vi "main(Test DQMH modules).bak.vi"() -> ()   [LabVIEW 2018, in "Application.lvlib"] (continued)
        n3308 = Bundle By Name(cluster=w7269, "command"="MEAS.eMIC", "command data"=w7266) -> (w7261:T11)
        n3309 = Bundle By Name(cluster=w7269, "command"="MEAS.AllRelaysOFF") -> (w7265:T11)
        n3310 = Build Array(w7265, w7264, w7263, w7262, w7261) -> (w7256:T11[])
        n3311 = Bundle By Name(cluster=w7243, "command"="MEAS.requestAC", "command data"=w7236) -> (w7257:T11)
        n3312 = Bundle By Name(cluster=w7243, "command"="Apps.WaitForEvent", "command data"=w7236) -> (w7242:T11)
        n3313 = Bundle By Name(cluster=w7243, "command"="MEAS.DMM dual read") -> (w7258:T11)
        n3314 = Bundle By Name(cluster=w7243, "command"="Apps.UI Update 1") -> (w7244:T11)
        n3315 = Build Array(w7258, w7257, w7242, w7244) -> (w7255:T11[])
        n3316 = Build Array (concatenate)(w7256, w7255) -> (w7254:T11[])
        n3317 = for {
          tunnel: w7254 -> [w7291] mode=indexing
          tunnel: w7249 -> [w7292]
          tunnel: [w7288] -> w7252 mode=indexing
          n3318 = Unbundle By Name(w7291) -> ("command"=w7290:string, "command data"=w7289:variant)
          n3319 = call "App enquece.vi"("command data"=w7289, "command"=w7290, "queue in"=w7292) -> ("error out"=w7288:errorcluster)  [unwired: 7 in, 1 out]
        }
        n3320 = Merge Errors(w7253, w7252) -> (w7251:errorcluster)
      }
      frame "Test DRV 29A" {
        w7300 = T11 {"command"="", "command data"=variant} ("element")
        w7294 = 29 ("DUT index(0-59)")
        w7326 = T11 {"command"="", "command data"=variant} ("element")
        n3321 = disable-structure shown="LOGGING==TRUE" {
          disable-tunnel: w7304 -> [w7341 _]
          frame condition #0 (active) {
            n3322 = Empty String/Path?(string/path=w7341) -> (empty?=w7344:bool)
            n3323 = Select(t="Quece timeout", s=w7344, f=w7341) -> (s? t:f=w7340:string)
            n3324 = call "string log (SubVI).vi"("Enum"=enum16{"Init", "Log", "Read"}."Log", "state Name"=w7340) -> ()  [unwired: 8 in, 2 out]
          }
          frame condition #1 {
          }
        }
        n3325 = Flush Queue(queue=w7305) -> (queue out=w7306:refnum<queue>)  [unwired: 1 in, 2 out]
        n3326 = Decrement(x=w7294) -> (x-1=w7297:i32)
        n3327 = Index Array(array=w7293, index=w7297) -> (element=w7295:refnum<vi>)
        n3328 = property class="ColBox"(reference=w7295, "Value"=u32 10000536 ("DRV 1")) -> ()  [unwired: 1 in, 2 out]
        n3329 = To Variant(anything=bool[] [FALSE, FALSE, FALSE, FALSE, TRUE, FALSE]) -> (Variant=w7323:variant)
        n3330 = To Variant(anything=T6."demux1_10_channel5" ("demux1_10(x6)_encode")) -> (Variant=w7327:variant)
        n3331 = To Variant(anything=T4."mux6_1_channel5_3" ("mux6_1(3wires)_encode")) -> (Variant=w7330:variant)
        n3332 = To Variant(anything=T5."mux10_1_channel5" ("mux10_1(x6)_encode")) -> (Variant=w7332:variant)
        n3333 = Bundle By Name(cluster=w7326, "command"="MEAS.mux10-1", "command data"=w7332) -> (w7321:T11)
        n3334 = Bundle By Name(cluster=w7326, "command"="MEAS.mux6_1", "command data"=w7330) -> (w7320:T11)
        n3335 = Bundle By Name(cluster=w7326, "command"="MEAS.demux1-10", "command data"=w7327) -> (w7319:T11)
        n3336 = Bundle By Name(cluster=w7326, "command"="MEAS.eMIC", "command data"=w7323) -> (w7318:T11)
        n3337 = Bundle By Name(cluster=w7326, "command"="MEAS.AllRelaysOFF") -> (w7322:T11)
        n3338 = Build Array(w7322, w7321, w7320, w7319, w7318) -> (w7313:T11[])
        n3339 = Bundle By Name(cluster=w7300, "command"="MEAS.requestAC", "command data"=w7294) -> (w7314:T11)
        n3340 = Bundle By Name(cluster=w7300, "command"="Apps.WaitForEvent", "command data"=w7294) -> (w7299:T11)
        n3341 = Bundle By Name(cluster=w7300, "command"="MEAS.DMM dual read") -> (w7315:T11)
        n3342 = Bundle By Name(cluster=w7300, "command"="Apps.UI Update 1") -> (w7301:T11)
        n3343 = Build Array(w7315, w7314, w7299, w7301) -> (w7312:T11[])
        n3344 = Build Array (concatenate)(w7313, w7312) -> (w7311:T11[])
        n3345 = for {
          tunnel: w7311 -> [w7348] mode=indexing
          tunnel: w7306 -> [w7349]
          tunnel: [w7345] -> w7309 mode=indexing
          n3346 = Unbundle By Name(w7348) -> ("command"=w7347:string, "command data"=w7346:variant)
          n3347 = call "App enquece.vi"("command data"=w7346, "command"=w7347, "queue in"=w7349) -> ("error out"=w7345:errorcluster)  [unwired: 7 in, 1 out]
        }
        n3348 = Merge Errors(w7310, w7309) -> (w7308:errorcluster)
      }
      frame "Test DRV 30A" {
        w7357 = T11 {"command"="", "command data"=variant} ("element")
        w7350 = 30 ("DUT index(0-59)")
        w7383 = T11 {"command"="", "command data"=variant} ("element")
        n3349 = disable-structure shown="LOGGING==TRUE" {
          disable-tunnel: w7361 -> [w7398 _]
          frame condition #0 (active) {
            n3350 = Empty String/Path?(string/path=w7398) -> (empty?=w7401:bool)
            n3351 = Select(t="Quece timeout", s=w7401, f=w7398) -> (s? t:f=w7397:string)
            n3352 = call "string log (SubVI).vi"("Enum"=enum16{"Init", "Log", "Read"}."Log", "state Name"=w7397) -> ()  [unwired: 8 in, 2 out]
          }
          frame condition #1 {
          }
        }
        n3353 = Flush Queue(queue=w7362) -> (queue out=w7363:refnum<queue>)  [unwired: 1 in, 2 out]
        n3354 = Decrement(x=w7350) -> (x-1=w7354:i32)
        n3355 = Index Array(array=w7351, index=w7354) -> (element=w7352:refnum<vi>)
        n3356 = property class="ColBox"(reference=w7352, "Value"=u32 10000536 ("DRV 1")) -> ()  [unwired: 1 in, 2 out]
        n3357 = To Variant(anything=bool[] [FALSE, FALSE, FALSE, FALSE, FALSE, TRUE]) -> (Variant=w7380:variant)
        n3358 = To Variant(anything=T6."demux1_10_channel5" ("demux1_10(x6)_encode")) -> (Variant=w7384:variant)
        n3359 = To Variant(anything=T4."mux6_1_channel6_3" ("mux6_1(3wires)_encode")) -> (Variant=w7387:variant)
        n3360 = To Variant(anything=T5."mux10_1_channel5" ("mux10_1(x6)_encode")) -> (Variant=w7389:variant)
        n3361 = Bundle By Name(cluster=w7383, "command"="MEAS.mux10-1", "command data"=w7389) -> (w7378:T11)
        n3362 = Bundle By Name(cluster=w7383, "command"="MEAS.mux6_1", "command data"=w7387) -> (w7377:T11)
        n3363 = Bundle By Name(cluster=w7383, "command"="MEAS.demux1-10", "command data"=w7384) -> (w7376:T11)
        n3364 = Bundle By Name(cluster=w7383, "command"="MEAS.eMIC", "command data"=w7380) -> (w7375:T11)
        n3365 = Bundle By Name(cluster=w7383, "command"="MEAS.AllRelaysOFF") -> (w7379:T11)
        n3366 = Build Array(w7379, w7378, w7377, w7376, w7375) -> (w7370:T11[])
        n3367 = Bundle By Name(cluster=w7357, "command"="MEAS.requestAC", "command data"=w7350) -> (w7371:T11)
        n3368 = Bundle By Name(cluster=w7357, "command"="Apps.WaitForEvent", "command data"=w7350) -> (w7356:T11)
        n3369 = Bundle By Name(cluster=w7357, "command"="MEAS.DMM dual read") -> (w7372:T11)
        n3370 = Bundle By Name(cluster=w7357, "command"="Apps.UI Update 1") -> (w7358:T11)
        n3371 = Build Array(w7372, w7371, w7356, w7358) -> (w7369:T11[])
        n3372 = Build Array (concatenate)(w7370, w7369) -> (w7368:T11[])
        n3373 = for {
          tunnel: w7368 -> [w7405] mode=indexing
          tunnel: w7363 -> [w7406]
          tunnel: [w7402] -> w7366 mode=indexing
          n3374 = Unbundle By Name(w7405) -> ("command"=w7404:string, "command data"=w7403:variant)
          n3375 = call "App enquece.vi"("command data"=w7403, "command"=w7404, "queue in"=w7406) -> ("error out"=w7402:errorcluster)  [unwired: 7 in, 1 out]
        }
        n3376 = Merge Errors(w7367, w7366) -> (w7365:errorcluster)
      }
      frame "Test DRV 31A" {
        w7414 = T11 {"command"="", "command data"=variant} ("element")
        w7407 = 31 ("DUT index(0-59)")
        w7440 = T11 {"command"="", "command data"=variant} ("element")
        n3377 = disable-structure shown="LOGGING==TRUE" {
          disable-tunnel: w7418 -> [w7455 _]
          frame condition #0 (active) {
            n3378 = Empty String/Path?(string/path=w7455) -> (empty?=w7458:bool)
            n3379 = Select(t="Quece timeout", s=w7458, f=w7455) -> (s? t:f=w7454:string)
            n3380 = call "string log (SubVI).vi"("Enum"=enum16{"Init", "Log", "Read"}."Log", "state Name"=w7454) -> ()  [unwired: 8 in, 2 out]
          }
          frame condition #1 {
          }
        }
        n3381 = Flush Queue(queue=w7419) -> (queue out=w7420:refnum<queue>)  [unwired: 1 in, 2 out]
        n3382 = Decrement(x=w7407) -> (x-1=w7411:i32)
        n3383 = Index Array(array=w7408, index=w7411) -> (element=w7409:refnum<vi>)
        n3384 = property class="ColBox"(reference=w7409, "Value"=u32 10000536 ("DRV 1")) -> ()  [unwired: 1 in, 2 out]
        n3385 = To Variant(anything=bool[] [TRUE, FALSE, FALSE, FALSE, FALSE, FALSE]) -> (Variant=w7437:variant)
        n3386 = To Variant(anything=T6."demux1_10_channel6" ("demux1_10(x6)_encode")) -> (Variant=w7441:variant)
        n3387 = To Variant(anything=T4."mux6_1_channel1_3" ("mux6_1(3wires)_encode")) -> (Variant=w7444:variant)
        n3388 = To Variant(anything=T5."mux10_1_channel6" ("mux10_1(x6)_encode")) -> (Variant=w7446:variant)
        n3389 = Bundle By Name(cluster=w7440, "command"="MEAS.mux10-1", "command data"=w7446) -> (w7435:T11)
        n3390 = Bundle By Name(cluster=w7440, "command"="MEAS.mux6_1", "command data"=w7444) -> (w7434:T11)
        n3391 = Bundle By Name(cluster=w7440, "command"="MEAS.demux1-10", "command data"=w7441) -> (w7433:T11)
        n3392 = Bundle By Name(cluster=w7440, "command"="MEAS.eMIC", "command data"=w7437) -> (w7432:T11)
        n3393 = Bundle By Name(cluster=w7440, "command"="MEAS.AllRelaysOFF") -> (w7436:T11)
        n3394 = Build Array(w7436, w7435, w7434, w7433, w7432) -> (w7427:T11[])
        n3395 = Bundle By Name(cluster=w7414, "command"="MEAS.requestAC", "command data"=w7407) -> (w7428:T11)
        n3396 = Bundle By Name(cluster=w7414, "command"="Apps.WaitForEvent", "command data"=w7407) -> (w7413:T11)
        n3397 = Bundle By Name(cluster=w7414, "command"="MEAS.DMM dual read") -> (w7429:T11)
        n3398 = Bundle By Name(cluster=w7414, "command"="Apps.UI Update 1") -> (w7415:T11)
        n3399 = Build Array(w7429, w7428, w7413, w7415) -> (w7426:T11[])
        n3400 = Build Array (concatenate)(w7427, w7426) -> (w7425:T11[])
        n3401 = for {
          tunnel: w7425 -> [w7462] mode=indexing
          tunnel: w7420 -> [w7463]
          tunnel: [w7459] -> w7423 mode=indexing
          n3402 = Unbundle By Name(w7462) -> ("command"=w7461:string, "command data"=w7460:variant)
          n3403 = call "App enquece.vi"("command data"=w7460, "command"=w7461, "queue in"=w7463) -> ("error out"=w7459:errorcluster)  [unwired: 7 in, 1 out]
        }
        n3404 = Merge Errors(w7424, w7423) -> (w7422:errorcluster)
      }
      frame "Test DRV 32A" {
        w7471 = T11 {"command"="", "command data"=variant} ("element")
        w7464 = 32 ("DUT index(0-59)")
        w7497 = T11 {"command"="", "command data"=variant} ("element")
        n3405 = disable-structure shown="LOGGING==TRUE" {
          disable-tunnel: w7475 -> [w7512 _]
          frame condition #0 (active) {
            n3406 = Empty String/Path?(string/path=w7512) -> (empty?=w7515:bool)
            n3407 = Select(t="Quece timeout", s=w7515, f=w7512) -> (s? t:f=w7511:string)
            n3408 = call "string log (SubVI).vi"("Enum"=enum16{"Init", "Log", "Read"}."Log", "state Name"=w7511) -> ()  [unwired: 8 in, 2 out]
          }
          frame condition #1 {
          }
        }
        n3409 = Flush Queue(queue=w7476) -> (queue out=w7477:refnum<queue>)  [unwired: 1 in, 2 out]
        n3410 = Decrement(x=w7464) -> (x-1=w7468:i32)
        n3411 = Index Array(array=w7465, index=w7468) -> (element=w7466:refnum<vi>)
        n3412 = property class="ColBox"(reference=w7466, "Value"=u32 10000536 ("DRV 1")) -> ()  [unwired: 1 in, 2 out]
        n3413 = To Variant(anything=bool[] [FALSE, TRUE, FALSE, FALSE, FALSE, FALSE]) -> (Variant=w7494:variant)
        n3414 = To Variant(anything=T6."demux1_10_channel6" ("demux1_10(x6)_encode")) -> (Variant=w7498:variant)
        n3415 = To Variant(anything=T4."mux6_1_channel2_3" ("mux6_1(3wires)_encode")) -> (Variant=w7501:variant)
        n3416 = To Variant(anything=T5."mux10_1_channel6" ("mux10_1(x6)_encode")) -> (Variant=w7503:variant)
        n3417 = Bundle By Name(cluster=w7497, "command"="MEAS.mux10-1", "command data"=w7503) -> (w7492:T11)
        n3418 = Bundle By Name(cluster=w7497, "command"="MEAS.mux6_1", "command data"=w7501) -> (w7491:T11)
        n3419 = Bundle By Name(cluster=w7497, "command"="MEAS.demux1-10", "command data"=w7498) -> (w7490:T11)
        n3420 = Bundle By Name(cluster=w7497, "command"="MEAS.eMIC", "command data"=w7494) -> (w7489:T11)
        n3421 = Bundle By Name(cluster=w7497, "command"="MEAS.AllRelaysOFF") -> (w7493:T11)
        n3422 = Build Array(w7493, w7492, w7491, w7490, w7489) -> (w7484:T11[])
        n3423 = Bundle By Name(cluster=w7471, "command"="MEAS.requestAC", "command data"=w7464) -> (w7485:T11)
        n3424 = Bundle By Name(cluster=w7471, "command"="Apps.WaitForEvent", "command data"=w7464) -> (w7470:T11)
        n3425 = Bundle By Name(cluster=w7471, "command"="MEAS.DMM dual read") -> (w7486:T11)
        n3426 = Bundle By Name(cluster=w7471, "command"="Apps.UI Update 1") -> (w7472:T11)
        n3427 = Build Array(w7486, w7485, w7470, w7472) -> (w7483:T11[])
        n3428 = Build Array (concatenate)(w7484, w7483) -> (w7482:T11[])
        n3429 = for {
          tunnel: w7482 -> [w7519] mode=indexing
          tunnel: w7477 -> [w7520]
          tunnel: [w7516] -> w7480 mode=indexing
          n3430 = Unbundle By Name(w7519) -> ("command"=w7518:string, "command data"=w7517:variant)
          n3431 = call "App enquece.vi"("command data"=w7517, "command"=w7518, "queue in"=w7520) -> ("error out"=w7516:errorcluster)  [unwired: 7 in, 1 out]
        }
        n3432 = Merge Errors(w7481, w7480) -> (w7479:errorcluster)
      }
      frame "Test DRV 33A" {
        w7528 = T11 {"command"="", "command data"=variant} ("element")
        w7522 = 33 ("DUT index(0-59)")
        w7554 = T11 {"command"="", "command data"=variant} ("element")
        n3433 = disable-structure shown="LOGGING==TRUE" {
          disable-tunnel: w7532 -> [w7569 _]
          frame condition #0 (active) {
            n3434 = Empty String/Path?(string/path=w7569) -> (empty?=w7572:bool)
            n3435 = Select(t="Quece timeout", s=w7572, f=w7569) -> (s? t:f=w7568:string)
            n3436 = call "string log (SubVI).vi"("Enum"=enum16{"Init", "Log", "Read"}."Log", "state Name"=w7568) -> ()  [unwired: 8 in, 2 out]
          }
          frame condition #1 {
          }
        }
        n3437 = Flush Queue(queue=w7533) -> (queue out=w7534:refnum<queue>)  [unwired: 1 in, 2 out]
        n3438 = Decrement(x=w7522) -> (x-1=w7525:i32)
        n3439 = Index Array(array=w7521, index=w7525) -> (element=w7523:refnum<vi>)
        n3440 = property class="ColBox"(reference=w7523, "Value"=u32 10000536 ("DRV 1")) -> ()  [unwired: 1 in, 2 out]
        n3441 = To Variant(anything=bool[] [FALSE, FALSE, TRUE, FALSE, FALSE, FALSE]) -> (Variant=w7551:variant)
        n3442 = To Variant(anything=T6."demux1_10_channel6" ("demux1_10(x6)_encode")) -> (Variant=w7555:variant)
        n3443 = To Variant(anything=T4."mux6_1_channel3_3" ("mux6_1(3wires)_encode")) -> (Variant=w7558:variant)
        n3444 = To Variant(anything=T5."mux10_1_channel6" ("mux10_1(x6)_encode")) -> (Variant=w7560:variant)
        n3445 = Bundle By Name(cluster=w7554, "command"="MEAS.mux10-1", "command data"=w7560) -> (w7549:T11)
        n3446 = Bundle By Name(cluster=w7554, "command"="MEAS.mux6_1", "command data"=w7558) -> (w7548:T11)
        n3447 = Bundle By Name(cluster=w7554, "command"="MEAS.demux1-10", "command data"=w7555) -> (w7547:T11)
        n3448 = Bundle By Name(cluster=w7554, "command"="MEAS.eMIC", "command data"=w7551) -> (w7546:T11)
        n3449 = Bundle By Name(cluster=w7554, "command"="MEAS.AllRelaysOFF") -> (w7550:T11)
        n3450 = Build Array(w7550, w7549, w7548, w7547, w7546) -> (w7541:T11[])
        n3451 = Bundle By Name(cluster=w7528, "command"="MEAS.requestAC", "command data"=w7522) -> (w7542:T11)
        n3452 = Bundle By Name(cluster=w7528, "command"="Apps.WaitForEvent", "command data"=w7522) -> (w7527:T11)
        n3453 = Bundle By Name(cluster=w7528, "command"="MEAS.DMM dual read") -> (w7543:T11)
        n3454 = Bundle By Name(cluster=w7528, "command"="Apps.UI Update 1") -> (w7529:T11)
        n3455 = Build Array(w7543, w7542, w7527, w7529) -> (w7540:T11[])
        n3456 = Build Array (concatenate)(w7541, w7540) -> (w7539:T11[])
        n3457 = for {
          tunnel: w7539 -> [w7576] mode=indexing
          tunnel: w7534 -> [w7577]
          tunnel: [w7573] -> w7537 mode=indexing
          n3458 = Unbundle By Name(w7576) -> ("command"=w7575:string, "command data"=w7574:variant)
          n3459 = call "App enquece.vi"("command data"=w7574, "command"=w7575, "queue in"=w7577) -> ("error out"=w7573:errorcluster)  [unwired: 7 in, 1 out]
        }
        n3460 = Merge Errors(w7538, w7537) -> (w7536:errorcluster)
      }
      frame "Test DRV 34A" {
        w7585 = T11 {"command"="", "command data"=variant} ("element")
        w7579 = 34 ("DUT index(0-59)")
        w7611 = T11 {"command"="", "command data"=variant} ("element")
        n3461 = disable-structure shown="LOGGING==TRUE" {
          disable-tunnel: w7589 -> [w7626 _]
          frame condition #0 (active) {
            n3462 = Empty String/Path?(string/path=w7626) -> (empty?=w7629:bool)
            n3463 = Select(t="Quece timeout", s=w7629, f=w7626) -> (s? t:f=w7625:string)
            n3464 = call "string log (SubVI).vi"("Enum"=enum16{"Init", "Log", "Read"}."Log", "state Name"=w7625) -> ()  [unwired: 8 in, 2 out]
          }
          frame condition #1 {
          }
        }
        n3465 = Flush Queue(queue=w7590) -> (queue out=w7591:refnum<queue>)  [unwired: 1 in, 2 out]
        n3466 = Decrement(x=w7579) -> (x-1=w7582:i32)
        n3467 = Index Array(array=w7578, index=w7582) -> (element=w7580:refnum<vi>)
        n3468 = property class="ColBox"(reference=w7580, "Value"=u32 10000536 ("DRV 1")) -> ()  [unwired: 1 in, 2 out]
        n3469 = To Variant(anything=bool[] [FALSE, FALSE, FALSE, TRUE, FALSE, FALSE]) -> (Variant=w7608:variant)
        n3470 = To Variant(anything=T6."demux1_10_channel6" ("demux1_10(x6)_encode")) -> (Variant=w7612:variant)
        n3471 = To Variant(anything=T4."mux6_1_channel4_3" ("mux6_1(3wires)_encode")) -> (Variant=w7615:variant)
        n3472 = To Variant(anything=T5."mux10_1_channel6" ("mux10_1(x6)_encode")) -> (Variant=w7617:variant)
        n3473 = Bundle By Name(cluster=w7611, "command"="MEAS.mux10-1", "command data"=w7617) -> (w7606:T11)
        n3474 = Bundle By Name(cluster=w7611, "command"="MEAS.mux6_1", "command data"=w7615) -> (w7605:T11)
        n3475 = Bundle By Name(cluster=w7611, "command"="MEAS.demux1-10", "command data"=w7612) -> (w7604:T11)
        n3476 = Bundle By Name(cluster=w7611, "command"="MEAS.eMIC", "command data"=w7608) -> (w7603:T11)
        n3477 = Bundle By Name(cluster=w7611, "command"="MEAS.AllRelaysOFF") -> (w7607:T11)
        n3478 = Build Array(w7607, w7606, w7605, w7604, w7603) -> (w7598:T11[])
        n3479 = Bundle By Name(cluster=w7585, "command"="MEAS.requestAC", "command data"=w7579) -> (w7599:T11)
        n3480 = Bundle By Name(cluster=w7585, "command"="Apps.WaitForEvent", "command data"=w7579) -> (w7584:T11)
        n3481 = Bundle By Name(cluster=w7585, "command"="MEAS.DMM dual read") -> (w7600:T11)
        n3482 = Bundle By Name(cluster=w7585, "command"="Apps.UI Update 1") -> (w7586:T11)
        n3483 = Build Array(w7600, w7599, w7584, w7586) -> (w7597:T11[])
        n3484 = Build Array (concatenate)(w7598, w7597) -> (w7596:T11[])
        n3485 = for {
          tunnel: w7596 -> [w7633] mode=indexing
          tunnel: w7591 -> [w7634]
          tunnel: [w7630] -> w7594 mode=indexing
          n3486 = Unbundle By Name(w7633) -> ("command"=w7632:string, "command data"=w7631:variant)
          n3487 = call "App enquece.vi"("command data"=w7631, "command"=w7632, "queue in"=w7634) -> ("error out"=w7630:errorcluster)  [unwired: 7 in, 1 out]
        }
        n3488 = Merge Errors(w7595, w7594) -> (w7593:errorcluster)
      }
      frame "Test DRV 35A" {
        w7642 = T11 {"command"="", "command data"=variant} ("element")
        w7635 = 35 ("DUT index(0-59)")
        w7668 = T11 {"command"="", "command data"=variant} ("element")
        n3489 = disable-structure shown="LOGGING==TRUE" {
          disable-tunnel: w7646 -> [w7683 _]
          frame condition #0 (active) {
            n3490 = Empty String/Path?(string/path=w7683) -> (empty?=w7686:bool)
            n3491 = Select(t="Quece timeout", s=w7686, f=w7683) -> (s? t:f=w7682:string)
            n3492 = call "string log (SubVI).vi"("Enum"=enum16{"Init", "Log", "Read"}."Log", "state Name"=w7682) -> ()  [unwired: 8 in, 2 out]
          }
          frame condition #1 {
          }
        }
        n3493 = Flush Queue(queue=w7647) -> (queue out=w7648:refnum<queue>)  [unwired: 1 in, 2 out]
        n3494 = Decrement(x=w7635) -> (x-1=w7639:i32)
        n3495 = Index Array(array=w7636, index=w7639) -> (element=w7637:refnum<vi>)
        n3496 = property class="ColBox"(reference=w7637, "Value"=u32 10000536 ("DRV 1")) -> ()  [unwired: 1 in, 2 out]
        n3497 = To Variant(anything=bool[] [FALSE, FALSE, FALSE, FALSE, TRUE, FALSE]) -> (Variant=w7665:variant)
        n3498 = To Variant(anything=T6."demux1_10_channel6" ("demux1_10(x6)_encode")) -> (Variant=w7669:variant)
        n3499 = To Variant(anything=T4."mux6_1_channel5_3" ("mux6_1(3wires)_encode")) -> (Variant=w7672:variant)
        n3500 = To Variant(anything=T5."mux10_1_channel6" ("mux10_1(x6)_encode")) -> (Variant=w7674:variant)
        n3501 = Bundle By Name(cluster=w7668, "command"="MEAS.mux10-1", "command data"=w7674) -> (w7663:T11)
        n3502 = Bundle By Name(cluster=w7668, "command"="MEAS.mux6_1", "command data"=w7672) -> (w7662:T11)
        n3503 = Bundle By Name(cluster=w7668, "command"="MEAS.demux1-10", "command data"=w7669) -> (w7661:T11)
        n3504 = Bundle By Name(cluster=w7668, "command"="MEAS.eMIC", "command data"=w7665) -> (w7660:T11)
        n3505 = Bundle By Name(cluster=w7668, "command"="MEAS.AllRelaysOFF") -> (w7664:T11)
        n3506 = Build Array(w7664, w7663, w7662, w7661, w7660) -> (w7655:T11[])
        n3507 = Bundle By Name(cluster=w7642, "command"="MEAS.requestAC", "command data"=w7635) -> (w7656:T11)
        n3508 = Bundle By Name(cluster=w7642, "command"="Apps.WaitForEvent", "command data"=w7635) -> (w7641:T11)
        n3509 = Bundle By Name(cluster=w7642, "command"="MEAS.DMM dual read") -> (w7657:T11)
        n3510 = Bundle By Name(cluster=w7642, "command"="Apps.UI Update 1") -> (w7643:T11)
        n3511 = Build Array(w7657, w7656, w7641, w7643) -> (w7654:T11[])
        n3512 = Build Array (concatenate)(w7655, w7654) -> (w7653:T11[])
        n3513 = for {
          tunnel: w7653 -> [w7690] mode=indexing
          tunnel: w7648 -> [w7691]
          tunnel: [w7687] -> w7651 mode=indexing
          n3514 = Unbundle By Name(w7690) -> ("command"=w7689:string, "command data"=w7688:variant)
          n3515 = call "App enquece.vi"("command data"=w7688, "command"=w7689, "queue in"=w7691) -> ("error out"=w7687:errorcluster)  [unwired: 7 in, 1 out]
        }
        n3516 = Merge Errors(w7652, w7651) -> (w7650:errorcluster)
      }
      frame "Test DRV 36A" {
        w7699 = T11 {"command"="", "command data"=variant} ("element")
        w7692 = 36 ("DUT index(0-59)")
        w7725 = T11 {"command"="", "command data"=variant} ("element")
        n3517 = disable-structure shown="LOGGING==TRUE" {
          disable-tunnel: w7703 -> [w7740 _]
          frame condition #0 (active) {
            n3518 = Empty String/Path?(string/path=w7740) -> (empty?=w7743:bool)
            n3519 = Select(t="Quece timeout", s=w7743, f=w7740) -> (s? t:f=w7739:string)
            n3520 = call "string log (SubVI).vi"("Enum"=enum16{"Init", "Log", "Read"}."Log", "state Name"=w7739) -> ()  [unwired: 8 in, 2 out]
          }
          frame condition #1 {
          }
        }
        n3521 = Flush Queue(queue=w7704) -> (queue out=w7705:refnum<queue>)  [unwired: 1 in, 2 out]
        n3522 = Decrement(x=w7692) -> (x-1=w7696:i32)
        n3523 = Index Array(array=w7693, index=w7696) -> (element=w7694:refnum<vi>)
        n3524 = property class="ColBox"(reference=w7694, "Value"=u32 10000536 ("DRV 1")) -> ()  [unwired: 1 in, 2 out]
        n3525 = To Variant(anything=bool[] [FALSE, FALSE, FALSE, FALSE, FALSE, TRUE]) -> (Variant=w7722:variant)
        n3526 = To Variant(anything=T6."demux1_10_channel6" ("demux1_10(x6)_encode")) -> (Variant=w7726:variant)
        n3527 = To Variant(anything=T4."mux6_1_channel6_3" ("mux6_1(3wires)_encode")) -> (Variant=w7729:variant)
        n3528 = To Variant(anything=T5."mux10_1_channel6" ("mux10_1(x6)_encode")) -> (Variant=w7731:variant)
        n3529 = Bundle By Name(cluster=w7725, "command"="MEAS.mux10-1", "command data"=w7731) -> (w7720:T11)
        n3530 = Bundle By Name(cluster=w7725, "command"="MEAS.mux6_1", "command data"=w7729) -> (w7719:T11)
        n3531 = Bundle By Name(cluster=w7725, "command"="MEAS.demux1-10", "command data"=w7726) -> (w7718:T11)
        n3532 = Bundle By Name(cluster=w7725, "command"="MEAS.eMIC", "command data"=w7722) -> (w7717:T11)
        n3533 = Bundle By Name(cluster=w7725, "command"="MEAS.AllRelaysOFF") -> (w7721:T11)
        n3534 = Build Array(w7721, w7720, w7719, w7718, w7717) -> (w7712:T11[])
        n3535 = Bundle By Name(cluster=w7699, "command"="MEAS.requestAC", "command data"=w7692) -> (w7713:T11)
        n3536 = Bundle By Name(cluster=w7699, "command"="Apps.WaitForEvent", "command data"=w7692) -> (w7698:T11)
        n3537 = Bundle By Name(cluster=w7699, "command"="MEAS.DMM dual read") -> (w7714:T11)
        n3538 = Bundle By Name(cluster=w7699, "command"="Apps.UI Update 1") -> (w7700:T11)
        n3539 = Build Array(w7714, w7713, w7698, w7700) -> (w7711:T11[])
        n3540 = Build Array (concatenate)(w7712, w7711) -> (w7710:T11[])
        n3541 = for {
          tunnel: w7710 -> [w7747] mode=indexing
          tunnel: w7705 -> [w7748]
          tunnel: [w7744] -> w7708 mode=indexing
          n3542 = Unbundle By Name(w7747) -> ("command"=w7746:string, "command data"=w7745:variant)
          n3543 = call "App enquece.vi"("command data"=w7745, "command"=w7746, "queue in"=w7748) -> ("error out"=w7744:errorcluster)  [unwired: 7 in, 1 out]
        }
        n3544 = Merge Errors(w7709, w7708) -> (w7707:errorcluster)
      }
      frame "Test DRV 37A" {
        w7756 = T11 {"command"="", "command data"=variant} ("element")
        w7749 = 37 ("DUT index(0-59)")
        w7782 = T11 {"command"="", "command data"=variant} ("element")
        n3545 = disable-structure shown="LOGGING==TRUE" {
          disable-tunnel: w7760 -> [w7797 _]
          frame condition #0 (active) {
            n3546 = Empty String/Path?(string/path=w7797) -> (empty?=w7800:bool)
            n3547 = Select(t="Quece timeout", s=w7800, f=w7797) -> (s? t:f=w7796:string)
            n3548 = call "string log (SubVI).vi"("Enum"=enum16{"Init", "Log", "Read"}."Log", "state Name"=w7796) -> ()  [unwired: 8 in, 2 out]
          }
          frame condition #1 {
          }
        }
        n3549 = Flush Queue(queue=w7761) -> (queue out=w7762:refnum<queue>)  [unwired: 1 in, 2 out]
        n3550 = Decrement(x=w7749) -> (x-1=w7753:i32)
        n3551 = Index Array(array=w7750, index=w7753) -> (element=w7751:refnum<vi>)
        n3552 = property class="ColBox"(reference=w7751, "Value"=u32 10000536 ("DRV 1")) -> ()  [unwired: 1 in, 2 out]
        n3553 = To Variant(anything=bool[] [TRUE, FALSE, FALSE, FALSE, FALSE, FALSE]) -> (Variant=w7779:variant)
        n3554 = To Variant(anything=T6."demux1_10_channel7" ("demux1_10(x6)_encode")) -> (Variant=w7783:variant)
        n3555 = To Variant(anything=T4."mux6_1_channel1_3" ("mux6_1(3wires)_encode")) -> (Variant=w7786:variant)
        n3556 = To Variant(anything=T5."mux10_1_channel7" ("mux10_1(x6)_encode")) -> (Variant=w7788:variant)
        n3557 = Bundle By Name(cluster=w7782, "command"="MEAS.mux10-1", "command data"=w7788) -> (w7777:T11)
        n3558 = Bundle By Name(cluster=w7782, "command"="MEAS.mux6_1", "command data"=w7786) -> (w7776:T11)
        n3559 = Bundle By Name(cluster=w7782, "command"="MEAS.demux1-10", "command data"=w7783) -> (w7775:T11)
        n3560 = Bundle By Name(cluster=w7782, "command"="MEAS.eMIC", "command data"=w7779) -> (w7774:T11)
        n3561 = Bundle By Name(cluster=w7782, "command"="MEAS.AllRelaysOFF") -> (w7778:T11)
        n3562 = Build Array(w7778, w7777, w7776, w7775, w7774) -> (w7769:T11[])
        n3563 = Bundle By Name(cluster=w7756, "command"="MEAS.requestAC", "command data"=w7749) -> (w7770:T11)
        n3564 = Bundle By Name(cluster=w7756, "command"="Apps.WaitForEvent", "command data"=w7749) -> (w7755:T11)
        n3565 = Bundle By Name(cluster=w7756, "command"="MEAS.DMM dual read") -> (w7771:T11)
        n3566 = Bundle By Name(cluster=w7756, "command"="Apps.UI Update 1") -> (w7757:T11)
        n3567 = Build Array(w7771, w7770, w7755, w7757) -> (w7768:T11[])
        n3568 = Build Array (concatenate)(w7769, w7768) -> (w7767:T11[])
        n3569 = for {
          tunnel: w7767 -> [w7804] mode=indexing
          tunnel: w7762 -> [w7805]
          tunnel: [w7801] -> w7765 mode=indexing
          n3570 = Unbundle By Name(w7804) -> ("command"=w7803:string, "command data"=w7802:variant)
          n3571 = call "App enquece.vi"("command data"=w7802, "command"=w7803, "queue in"=w7805) -> ("error out"=w7801:errorcluster)  [unwired: 7 in, 1 out]
        }
        n3572 = Merge Errors(w7766, w7765) -> (w7764:errorcluster)
      }
      frame "Test DRV 38A" {
        w7814 = T11 {"command"="", "command data"=variant} ("element")
        w7806 = 38 ("DUT index(0-59)")
        w7839 = T11 {"command"="", "command data"=variant} ("element")
        n3573 = disable-structure shown="LOGGING==TRUE" {
          disable-tunnel: w7818 -> [w7854 _]
          frame condition #0 (active) {
            n3574 = Empty String/Path?(string/path=w7854) -> (empty?=w7857:bool)
            n3575 = Select(t="Quece timeout", s=w7857, f=w7854) -> (s? t:f=w7853:string)
            n3576 = call "string log (SubVI).vi"("Enum"=enum16{"Init", "Log", "Read"}."Log", "state Name"=w7853) -> ()  [unwired: 8 in, 2 out]
          }
          frame condition #1 {
          }
        }
        n3577 = Flush Queue(queue=w7819) -> (queue out=w7811:refnum<queue>)  [unwired: 1 in, 2 out]
        n3578 = Decrement(x=w7806) -> (x-1=w7810:i32)
        n3579 = Index Array(array=w7807, index=w7810) -> (element=w7808:refnum<vi>)
        n3580 = property class="ColBox"(reference=w7808, "Value"=u32 10000536 ("DRV 1")) -> ()  [unwired: 1 in, 2 out]
        n3581 = To Variant(anything=bool[] [FALSE, TRUE, FALSE, FALSE, FALSE, FALSE]) -> (Variant=w7836:variant)
        n3582 = To Variant(anything=T6."demux1_10_channel7" ("demux1_10(x6)_encode")) -> (Variant=w7840:variant)
        n3583 = To Variant(anything=T4."mux6_1_channel2_3" ("mux6_1(3wires)_encode")) -> (Variant=w7843:variant)
        n3584 = To Variant(anything=T5."mux10_1_channel7" ("mux10_1(x6)_encode")) -> (Variant=w7845:variant)
        n3585 = Bundle By Name(cluster=w7839, "command"="MEAS.mux10-1", "command data"=w7845) -> (w7834:T11)
        n3586 = Bundle By Name(cluster=w7839, "command"="MEAS.mux6_1", "command data"=w7843) -> (w7833:T11)
        n3587 = Bundle By Name(cluster=w7839, "command"="MEAS.demux1-10", "command data"=w7840) -> (w7832:T11)
        n3588 = Bundle By Name(cluster=w7839, "command"="MEAS.eMIC", "command data"=w7836) -> (w7831:T11)
        n3589 = Bundle By Name(cluster=w7839, "command"="MEAS.AllRelaysOFF") -> (w7835:T11)
        n3590 = Build Array(w7835, w7834, w7833, w7832, w7831) -> (w7826:T11[])
        n3591 = Bundle By Name(cluster=w7814, "command"="MEAS.requestAC", "command data"=w7806) -> (w7827:T11)
        n3592 = Bundle By Name(cluster=w7814, "command"="Apps.WaitForEvent", "command data"=w7806) -> (w7813:T11)
        n3593 = Bundle By Name(cluster=w7814, "command"="MEAS.DMM dual read") -> (w7828:T11)
        n3594 = Bundle By Name(cluster=w7814, "command"="Apps.UI Update 1") -> (w7815:T11)
        n3595 = Build Array(w7828, w7827, w7813, w7815) -> (w7825:T11[])
        n3596 = Build Array (concatenate)(w7826, w7825) -> (w7824:T11[])
        n3597 = for {
          tunnel: w7824 -> [w7861] mode=indexing
          tunnel: w7811 -> [w7862]
          tunnel: [w7858] -> w7822 mode=indexing
          n3598 = Unbundle By Name(w7861) -> ("command"=w7860:string, "command data"=w7859:variant)
          n3599 = call "App enquece.vi"("command data"=w7859, "command"=w7860, "queue in"=w7862) -> ("error out"=w7858:errorcluster)  [unwired: 7 in, 1 out]
        }
        n3600 = Merge Errors(w7823, w7822) -> (w7821:errorcluster)
      }
      frame "Test DRV 39A" {
        w7870 = T11 {"command"="", "command data"=variant} ("element")
        w7863 = 39 ("DUT index(0-59)")
        w7896 = T11 {"command"="", "command data"=variant} ("element")
        n3601 = disable-structure shown="LOGGING==TRUE" {
          disable-tunnel: w7874 -> [w7911 _]
          frame condition #0 (active) {
            n3602 = Empty String/Path?(string/path=w7911) -> (empty?=w7914:bool)
            n3603 = Select(t="Quece timeout", s=w7914, f=w7911) -> (s? t:f=w7910:string)
            n3604 = call "string log (SubVI).vi"("Enum"=enum16{"Init", "Log", "Read"}."Log", "state Name"=w7910) -> ()  [unwired: 8 in, 2 out]
          }
          frame condition #1 {
          }
        }
        n3605 = Flush Queue(queue=w7875) -> (queue out=w7876:refnum<queue>)  [unwired: 1 in, 2 out]
        n3606 = Decrement(x=w7863) -> (x-1=w7867:i32)
        n3607 = Index Array(array=w7864, index=w7867) -> (element=w7865:refnum<vi>)
        n3608 = property class="ColBox"(reference=w7865, "Value"=u32 10000536 ("DRV 1")) -> ()  [unwired: 1 in, 2 out]
        n3609 = To Variant(anything=bool[] [FALSE, FALSE, TRUE, FALSE, FALSE, FALSE]) -> (Variant=w7893:variant)
        n3610 = To Variant(anything=T6."demux1_10_channel7" ("demux1_10(x6)_encode")) -> (Variant=w7897:variant)
        n3611 = To Variant(anything=T4."mux6_1_channel3_3" ("mux6_1(3wires)_encode")) -> (Variant=w7900:variant)
        n3612 = To Variant(anything=T5."mux10_1_channel7" ("mux10_1(x6)_encode")) -> (Variant=w7902:variant)
        n3613 = Bundle By Name(cluster=w7896, "command"="MEAS.mux10-1", "command data"=w7902) -> (w7891:T11)
        n3614 = Bundle By Name(cluster=w7896, "command"="MEAS.mux6_1", "command data"=w7900) -> (w7890:T11)
        n3615 = Bundle By Name(cluster=w7896, "command"="MEAS.demux1-10", "command data"=w7897) -> (w7889:T11)
        n3616 = Bundle By Name(cluster=w7896, "command"="MEAS.eMIC", "command data"=w7893) -> (w7888:T11)
        n3617 = Bundle By Name(cluster=w7896, "command"="MEAS.AllRelaysOFF") -> (w7892:T11)
        n3618 = Build Array(w7892, w7891, w7890, w7889, w7888) -> (w7883:T11[])
        n3619 = Bundle By Name(cluster=w7870, "command"="MEAS.requestAC", "command data"=w7863) -> (w7884:T11)
        n3620 = Bundle By Name(cluster=w7870, "command"="Apps.WaitForEvent", "command data"=w7863) -> (w7869:T11)
        n3621 = Bundle By Name(cluster=w7870, "command"="MEAS.DMM dual read") -> (w7885:T11)
        n3622 = Bundle By Name(cluster=w7870, "command"="Apps.UI Update 1") -> (w7871:T11)
        n3623 = Build Array(w7885, w7884, w7869, w7871) -> (w7882:T11[])
        n3624 = Build Array (concatenate)(w7883, w7882) -> (w7881:T11[])
        n3625 = for {
          tunnel: w7881 -> [w7918] mode=indexing
          tunnel: w7876 -> [w7919]
          tunnel: [w7915] -> w7879 mode=indexing
          n3626 = Unbundle By Name(w7918) -> ("command"=w7917:string, "command data"=w7916:variant)
          n3627 = call "App enquece.vi"("command data"=w7916, "command"=w7917, "queue in"=w7919) -> ("error out"=w7915:errorcluster)  [unwired: 7 in, 1 out]
        }
        n3628 = Merge Errors(w7880, w7879) -> (w7878:errorcluster)
      }
      frame "Test DRV 40A" {
        w7927 = T11 {"command"="", "command data"=variant} ("element")
        w7920 = 40 ("DUT index(0-59)")
        w7953 = T11 {"command"="", "command data"=variant} ("element")
        n3629 = disable-structure shown="LOGGING==TRUE" {
          disable-tunnel: w7931 -> [w7968 _]
          frame condition #0 (active) {
            n3630 = Empty String/Path?(string/path=w7968) -> (empty?=w7971:bool)
            n3631 = Select(t="Quece timeout", s=w7971, f=w7968) -> (s? t:f=w7967:string)
            n3632 = call "string log (SubVI).vi"("Enum"=enum16{"Init", "Log", "Read"}."Log", "state Name"=w7967) -> ()  [unwired: 8 in, 2 out]
          }
          frame condition #1 {
          }
        }
        n3633 = Flush Queue(queue=w7932) -> (queue out=w7933:refnum<queue>)  [unwired: 1 in, 2 out]
        n3634 = Decrement(x=w7920) -> (x-1=w7924:i32)
        n3635 = Index Array(array=w7921, index=w7924) -> (element=w7922:refnum<vi>)
        n3636 = property class="ColBox"(reference=w7922, "Value"=u32 10000536 ("DRV 1")) -> ()  [unwired: 1 in, 2 out]
        n3637 = To Variant(anything=bool[] [FALSE, FALSE, FALSE, TRUE, FALSE, FALSE]) -> (Variant=w7950:variant)
        n3638 = To Variant(anything=T6."demux1_10_channel7" ("demux1_10(x6)_encode")) -> (Variant=w7954:variant)
        n3639 = To Variant(anything=T4."mux6_1_channel4_3" ("mux6_1(3wires)_encode")) -> (Variant=w7957:variant)
        n3640 = To Variant(anything=T5."mux10_1_channel7" ("mux10_1(x6)_encode")) -> (Variant=w7959:variant)
        n3641 = Bundle By Name(cluster=w7953, "command"="MEAS.mux10-1", "command data"=w7959) -> (w7948:T11)
        n3642 = Bundle By Name(cluster=w7953, "command"="MEAS.mux6_1", "command data"=w7957) -> (w7947:T11)
        n3643 = Bundle By Name(cluster=w7953, "command"="MEAS.demux1-10", "command data"=w7954) -> (w7946:T11)
        n3644 = Bundle By Name(cluster=w7953, "command"="MEAS.eMIC", "command data"=w7950) -> (w7945:T11)
        n3645 = Bundle By Name(cluster=w7953, "command"="MEAS.AllRelaysOFF") -> (w7949:T11)
        n3646 = Build Array(w7949, w7948, w7947, w7946, w7945) -> (w7940:T11[])
        n3647 = Bundle By Name(cluster=w7927, "command"="MEAS.requestAC", "command data"=w7920) -> (w7941:T11)
        n3648 = Bundle By Name(cluster=w7927, "command"="Apps.WaitForEvent", "command data"=w7920) -> (w7926:T11)
        n3649 = Bundle By Name(cluster=w7927, "command"="MEAS.DMM dual read") -> (w7942:T11)
        n3650 = Bundle By Name(cluster=w7927, "command"="Apps.UI Update 1") -> (w7928:T11)
        n3651 = Build Array(w7942, w7941, w7926, w7928) -> (w7939:T11[])
        n3652 = Build Array (concatenate)(w7940, w7939) -> (w7938:T11[])
        n3653 = for {
          tunnel: w7938 -> [w7975] mode=indexing
          tunnel: w7933 -> [w7976]
          tunnel: [w7972] -> w7936 mode=indexing
          n3654 = Unbundle By Name(w7975) -> ("command"=w7974:string, "command data"=w7973:variant)
          n3655 = call "App enquece.vi"("command data"=w7973, "command"=w7974, "queue in"=w7976) -> ("error out"=w7972:errorcluster)  [unwired: 7 in, 1 out]
        }
        n3656 = Merge Errors(w7937, w7936) -> (w7935:errorcluster)
      }
      frame "Test DRV 41A" {
        w7984 = T11 {"command"="", "command data"=variant} ("element")
        w7977 = 41 ("DUT index(0-59)")
        w8010 = T11 {"command"="", "command data"=variant} ("element")
        n3657 = disable-structure shown="LOGGING==TRUE" {
          disable-tunnel: w7988 -> [w8025 _]
          frame condition #0 (active) {
            n3658 = Empty String/Path?(string/path=w8025) -> (empty?=w8028:bool)
            n3659 = Select(t="Quece timeout", s=w8028, f=w8025) -> (s? t:f=w8024:string)
            n3660 = call "string log (SubVI).vi"("Enum"=enum16{"Init", "Log", "Read"}."Log", "state Name"=w8024) -> ()  [unwired: 8 in, 2 out]
          }
          frame condition #1 {
          }
        }
        n3661 = Flush Queue(queue=w7989) -> (queue out=w7990:refnum<queue>)  [unwired: 1 in, 2 out]
        n3662 = Decrement(x=w7977) -> (x-1=w7981:i32)
        n3663 = Index Array(array=w7978, index=w7981) -> (element=w7979:refnum<vi>)
        n3664 = property class="ColBox"(reference=w7979, "Value"=u32 10000536 ("DRV 1")) -> ()  [unwired: 1 in, 2 out]
        n3665 = To Variant(anything=bool[] [FALSE, FALSE, FALSE, FALSE, TRUE, FALSE]) -> (Variant=w8007:variant)
        n3666 = To Variant(anything=T6."demux1_10_channel7" ("demux1_10(x6)_encode")) -> (Variant=w8011:variant)
        n3667 = To Variant(anything=T4."mux6_1_channel5_3" ("mux6_1(3wires)_encode")) -> (Variant=w8014:variant)
        n3668 = To Variant(anything=T5."mux10_1_channel7" ("mux10_1(x6)_encode")) -> (Variant=w8016:variant)
        n3669 = Bundle By Name(cluster=w8010, "command"="MEAS.mux10-1", "command data"=w8016) -> (w8005:T11)
        n3670 = Bundle By Name(cluster=w8010, "command"="MEAS.mux6_1", "command data"=w8014) -> (w8004:T11)
        n3671 = Bundle By Name(cluster=w8010, "command"="MEAS.demux1-10", "command data"=w8011) -> (w8003:T11)
        n3672 = Bundle By Name(cluster=w8010, "command"="MEAS.eMIC", "command data"=w8007) -> (w8002:T11)
        n3673 = Bundle By Name(cluster=w8010, "command"="MEAS.AllRelaysOFF") -> (w8006:T11)
        n3674 = Build Array(w8006, w8005, w8004, w8003, w8002) -> (w7997:T11[])
        n3675 = Bundle By Name(cluster=w7984, "command"="MEAS.requestAC", "command data"=w7977) -> (w7998:T11)
        n3676 = Bundle By Name(cluster=w7984, "command"="Apps.WaitForEvent", "command data"=w7977) -> (w7983:T11)
        n3677 = Bundle By Name(cluster=w7984, "command"="MEAS.DMM dual read") -> (w7999:T11)
        n3678 = Bundle By Name(cluster=w7984, "command"="Apps.UI Update 1") -> (w7985:T11)
        n3679 = Build Array(w7999, w7998, w7983, w7985) -> (w7996:T11[])
        n3680 = Build Array (concatenate)(w7997, w7996) -> (w7995:T11[])
        n3681 = for {
          tunnel: w7995 -> [w8032] mode=indexing
          tunnel: w7990 -> [w8033]
          tunnel: [w8029] -> w7993 mode=indexing
          n3682 = Unbundle By Name(w8032) -> ("command"=w8031:string, "command data"=w8030:variant)
          n3683 = call "App enquece.vi"("command data"=w8030, "command"=w8031, "queue in"=w8033) -> ("error out"=w8029:errorcluster)  [unwired: 7 in, 1 out]
        }
        n3684 = Merge Errors(w7994, w7993) -> (w7992:errorcluster)
      }
      frame "Test DRV 42A" {
        w8041 = T11 {"command"="", "command data"=variant} ("element")
        w8034 = 42 ("DUT index(0-59)")
        w8067 = T11 {"command"="", "command data"=variant} ("element")
        n3685 = disable-structure shown="LOGGING==TRUE" {
          disable-tunnel: w8045 -> [w8082 _]
          frame condition #0 (active) {
            n3686 = Empty String/Path?(string/path=w8082) -> (empty?=w8085:bool)
            n3687 = Select(t="Quece timeout", s=w8085, f=w8082) -> (s? t:f=w8081:string)
            n3688 = call "string log (SubVI).vi"("Enum"=enum16{"Init", "Log", "Read"}."Log", "state Name"=w8081) -> ()  [unwired: 8 in, 2 out]
          }
          frame condition #1 {
          }
        }
        n3689 = Flush Queue(queue=w8046) -> (queue out=w8047:refnum<queue>)  [unwired: 1 in, 2 out]
        n3690 = Decrement(x=w8034) -> (x-1=w8038:i32)
        n3691 = Index Array(array=w8035, index=w8038) -> (element=w8036:refnum<vi>)
        n3692 = property class="ColBox"(reference=w8036, "Value"=u32 10000536 ("DRV 1")) -> ()  [unwired: 1 in, 2 out]
        n3693 = To Variant(anything=bool[] [FALSE, FALSE, FALSE, FALSE, FALSE, TRUE]) -> (Variant=w8064:variant)
        n3694 = To Variant(anything=T6."demux1_10_channel7" ("demux1_10(x6)_encode")) -> (Variant=w8068:variant)
        n3695 = To Variant(anything=T4."mux6_1_channel6_3" ("mux6_1(3wires)_encode")) -> (Variant=w8071:variant)
        n3696 = To Variant(anything=T5."mux10_1_channel7" ("mux10_1(x6)_encode")) -> (Variant=w8073:variant)
        n3697 = Bundle By Name(cluster=w8067, "command"="MEAS.mux10-1", "command data"=w8073) -> (w8062:T11)
        n3698 = Bundle By Name(cluster=w8067, "command"="MEAS.mux6_1", "command data"=w8071) -> (w8061:T11)
        n3699 = Bundle By Name(cluster=w8067, "command"="MEAS.demux1-10", "command data"=w8068) -> (w8060:T11)
        n3700 = Bundle By Name(cluster=w8067, "command"="MEAS.eMIC", "command data"=w8064) -> (w8059:T11)
        n3701 = Bundle By Name(cluster=w8067, "command"="MEAS.AllRelaysOFF") -> (w8063:T11)
        n3702 = Build Array(w8063, w8062, w8061, w8060, w8059) -> (w8054:T11[])
        n3703 = Bundle By Name(cluster=w8041, "command"="MEAS.requestAC", "command data"=w8034) -> (w8055:T11)
        n3704 = Bundle By Name(cluster=w8041, "command"="Apps.WaitForEvent", "command data"=w8034) -> (w8040:T11)
        n3705 = Bundle By Name(cluster=w8041, "command"="MEAS.DMM dual read") -> (w8056:T11)
        n3706 = Bundle By Name(cluster=w8041, "command"="Apps.UI Update 1") -> (w8042:T11)
        n3707 = Build Array(w8056, w8055, w8040, w8042) -> (w8053:T11[])
        n3708 = Build Array (concatenate)(w8054, w8053) -> (w8052:T11[])
        n3709 = for {
          tunnel: w8052 -> [w8089] mode=indexing
          tunnel: w8047 -> [w8090]
          tunnel: [w8086] -> w8050 mode=indexing
          n3710 = Unbundle By Name(w8089) -> ("command"=w8088:string, "command data"=w8087:variant)
          n3711 = call "App enquece.vi"("command data"=w8087, "command"=w8088, "queue in"=w8090) -> ("error out"=w8086:errorcluster)  [unwired: 7 in, 1 out]
        }
        n3712 = Merge Errors(w8051, w8050) -> (w8049:errorcluster)
      }
      frame "Test DRV 43A" {
        w8098 = T11 {"command"="", "command data"=variant} ("element")
        w8091 = 43 ("DUT index(0-59)")
        w8124 = T11 {"command"="", "command data"=variant} ("element")
        n3713 = disable-structure shown="LOGGING==TRUE" {
          disable-tunnel: w8102 -> [w8139 _]
          frame condition #0 (active) {
            n3714 = Empty String/Path?(string/path=w8139) -> (empty?=w8142:bool)
            n3715 = Select(t="Quece timeout", s=w8142, f=w8139) -> (s? t:f=w8138:string)
            n3716 = call "string log (SubVI).vi"("Enum"=enum16{"Init", "Log", "Read"}."Log", "state Name"=w8138) -> ()  [unwired: 8 in, 2 out]
          }
          frame condition #1 {
          }
        }
        n3717 = Flush Queue(queue=w8103) -> (queue out=w8104:refnum<queue>)  [unwired: 1 in, 2 out]
        n3718 = Decrement(x=w8091) -> (x-1=w8095:i32)
        n3719 = Index Array(array=w8092, index=w8095) -> (element=w8093:refnum<vi>)
        n3720 = property class="ColBox"(reference=w8093, "Value"=u32 10000536 ("DRV 1")) -> ()  [unwired: 1 in, 2 out]
        n3721 = To Variant(anything=bool[] [TRUE, FALSE, FALSE, FALSE, FALSE, FALSE]) -> (Variant=w8121:variant)
        n3722 = To Variant(anything=T6."demux1_10_channel8" ("demux1_10(x6)_encode")) -> (Variant=w8125:variant)
        n3723 = To Variant(anything=T4."mux6_1_channel1_3" ("mux6_1(3wires)_encode")) -> (Variant=w8128:variant)
        n3724 = To Variant(anything=T5."mux10_1_channel8" ("mux10_1(x6)_encode")) -> (Variant=w8130:variant)
        n3725 = Bundle By Name(cluster=w8124, "command"="MEAS.mux10-1", "command data"=w8130) -> (w8119:T11)
        n3726 = Bundle By Name(cluster=w8124, "command"="MEAS.mux6_1", "command data"=w8128) -> (w8118:T11)
        n3727 = Bundle By Name(cluster=w8124, "command"="MEAS.demux1-10", "command data"=w8125) -> (w8117:T11)
        n3728 = Bundle By Name(cluster=w8124, "command"="MEAS.eMIC", "command data"=w8121) -> (w8116:T11)
        n3729 = Bundle By Name(cluster=w8124, "command"="MEAS.AllRelaysOFF") -> (w8120:T11)
        n3730 = Build Array(w8120, w8119, w8118, w8117, w8116) -> (w8111:T11[])
        n3731 = Bundle By Name(cluster=w8098, "command"="MEAS.requestAC", "command data"=w8091) -> (w8112:T11)
        n3732 = Bundle By Name(cluster=w8098, "command"="Apps.WaitForEvent", "command data"=w8091) -> (w8097:T11)
        n3733 = Bundle By Name(cluster=w8098, "command"="MEAS.DMM dual read") -> (w8113:T11)
        n3734 = Bundle By Name(cluster=w8098, "command"="Apps.UI Update 1") -> (w8099:T11)
        n3735 = Build Array(w8113, w8112, w8097, w8099) -> (w8110:T11[])
        n3736 = Build Array (concatenate)(w8111, w8110) -> (w8109:T11[])
        n3737 = for {
          tunnel: w8109 -> [w8146] mode=indexing
          tunnel: w8104 -> [w8147]
          tunnel: [w8143] -> w8107 mode=indexing
          n3738 = Unbundle By Name(w8146) -> ("command"=w8145:string, "command data"=w8144:variant)
          n3739 = call "App enquece.vi"("command data"=w8144, "command"=w8145, "queue in"=w8147) -> ("error out"=w8143:errorcluster)  [unwired: 7 in, 1 out]
        }
        n3740 = Merge Errors(w8108, w8107) -> (w8106:errorcluster)
      }
      frame "Test DRV 44A" {
        w8155 = T11 {"command"="", "command data"=variant} ("element")
        w8151 = 44 ("DUT index(0-59)")
        w8181 = T11 {"command"="", "command data"=variant} ("element")
        n3741 = disable-structure shown="LOGGING==TRUE" {
          disable-tunnel: w8159 -> [w8196 _]
          frame condition #0 (active) {
            n3742 = Empty String/Path?(string/path=w8196) -> (empty?=w8199:bool)
            n3743 = Select(t="Quece timeout", s=w8199, f=w8196) -> (s? t:f=w8195:string)
            n3744 = call "string log (SubVI).vi"("Enum"=enum16{"Init", "Log", "Read"}."Log", "state Name"=w8195) -> ()  [unwired: 8 in, 2 out]
          }
          frame condition #1 {
          }
        }
        n3745 = Flush Queue(queue=w8160) -> (queue out=w8161:refnum<queue>)  [unwired: 1 in, 2 out]
        n3746 = Decrement(x=w8151) -> (x-1=w8152:i32)
        n3747 = Index Array(array=w8150, index=w8152) -> (element=w8148:refnum<vi>)
        n3748 = property class="ColBox"(reference=w8148, "Value"=u32 10000536 ("DRV 1")) -> ()  [unwired: 1 in, 2 out]
        n3749 = To Variant(anything=bool[] [FALSE, TRUE, FALSE, FALSE, FALSE, FALSE]) -> (Variant=w8178:variant)
        n3750 = To Variant(anything=T6."demux1_10_channel8" ("demux1_10(x6)_encode")) -> (Variant=w8182:variant)
        n3751 = To Variant(anything=T4."mux6_1_channel2_3" ("mux6_1(3wires)_encode")) -> (Variant=w8185:variant)
        n3752 = To Variant(anything=T5."mux10_1_channel8" ("mux10_1(x6)_encode")) -> (Variant=w8187:variant)
        n3753 = Bundle By Name(cluster=w8181, "command"="MEAS.mux10-1", "command data"=w8187) -> (w8176:T11)
        n3754 = Bundle By Name(cluster=w8181, "command"="MEAS.mux6_1", "command data"=w8185) -> (w8175:T11)
        n3755 = Bundle By Name(cluster=w8181, "command"="MEAS.demux1-10", "command data"=w8182) -> (w8174:T11)
        n3756 = Bundle By Name(cluster=w8181, "command"="MEAS.eMIC", "command data"=w8178) -> (w8173:T11)
        n3757 = Bundle By Name(cluster=w8181, "command"="MEAS.AllRelaysOFF") -> (w8177:T11)
        n3758 = Build Array(w8177, w8176, w8175, w8174, w8173) -> (w8168:T11[])
        n3759 = Bundle By Name(cluster=w8155, "command"="MEAS.requestAC", "command data"=w8151) -> (w8169:T11)
        n3760 = Bundle By Name(cluster=w8155, "command"="Apps.WaitForEvent", "command data"=w8151) -> (w8154:T11)
        n3761 = Bundle By Name(cluster=w8155, "command"="MEAS.DMM dual read") -> (w8170:T11)
        n3762 = Bundle By Name(cluster=w8155, "command"="Apps.UI Update 1") -> (w8156:T11)
        n3763 = Build Array(w8170, w8169, w8154, w8156) -> (w8167:T11[])
        n3764 = Build Array (concatenate)(w8168, w8167) -> (w8166:T11[])
        n3765 = for {
